vi "Parse Tag Header.vi"(11 "Tag Header String":string) -> (0 "</ Tag>":bool, 1 "Tag Name":string, 2 "Attr Vals":string[](array[string]), 3 "Attr Names":string[](array[string]))   [LabVIEW 2020, in "NI_VIAnCFGDataStructure.lvlib" / "Tree.lvclass"]
uses:
  <vilib>/addons/analyzer/VIAnCFGDataStructure/Tree Manager/Tree.lvclass
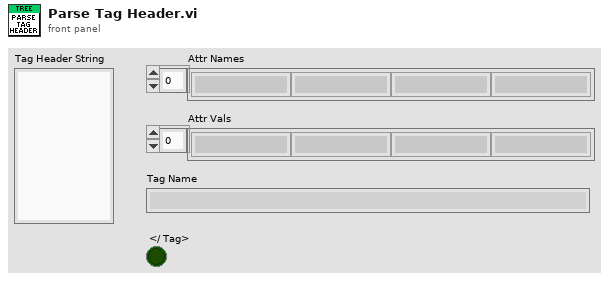
[diagram p1: front panel]
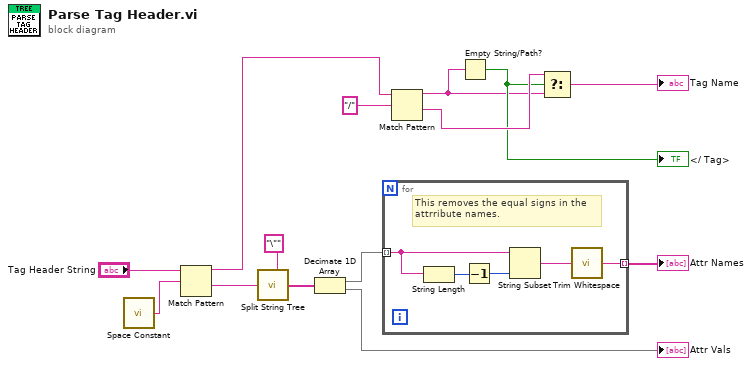
[diagram p0: block diagram]
diagram:
  n1 = call <vilib>:"Space Constant.vi"() -> ("String"=w10:string)
  n2 = Match Pattern(string="Tag Header String", regular expression=w10) -> (before substring=w9:string, after substring=w7:string)  [unwired: 1 in, 2 out]
  n3 = call <vilib>:"Split String Tree.vi"("Split Pattern"="\"", "Input String"=w7) -> ("Split String"=w6:string[])  [unwired: 5 in]
  n4 = Decimate 1D Array(w6) -> (w5:string[], →"Attr Vals":string[])
  n5 = for {
    tunnel: w5 -> [w17] mode=indexing
    tunnel: [w18] -> w3 mode=indexing
    # "This removes the equal signs in the\nattrribute names."
    n6 = String Length(string=w17) -> (length=w16:i32)
    n7 = Decrement(x=w16) -> (x-1=w15:i32)
    n8 = String Subset(string=w17, length (rest)=w15) -> (substring=w19:string)  [unwired: 1 in]
    n9 = call <vilib>:"Trim Whitespace.vi"("string"=w19) -> ("trimmed string"=w18:string)  [unwired: 1 in]
  }
  "Attr Names" <- w3
  n10 = Match Pattern(string=w9, regular expression="/") -> (before substring=w1:string, after substring=w12:string)  [unwired: 1 in, 2 out]
  n11 = Empty String/Path?(string/path=w1) -> (empty?=w2:bool)
  "</ Tag>" <- w2
  n12 = Select(t=w12, s=w2, f=w1) -> (s? t:f=→"Tag Name":string)
